vi "Channel List to Pins.vi"(0 "Channel List":string) -> (4 "Sites and Pins":string[](array[string]), 6 "Pins":tag[](array[tag]), 8 "Sites":i32[](array[numeric]))   [LabVIEW 2019]
uses:
  <vilib>/Utility/error.llb/whitespace.ctl
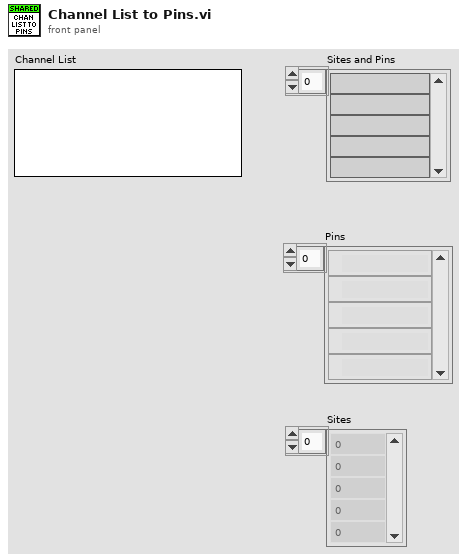
[diagram p1: front panel]
types:
  T1 = typedef "whitespace.ctl" = u16
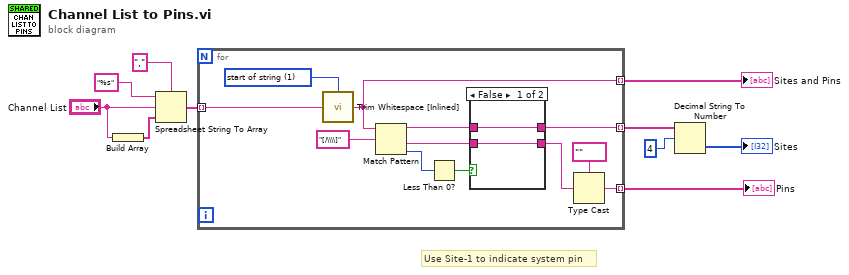
[diagram p0: block diagram]
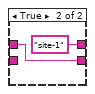
[diagram p2: hidden frame]
diagram:
  # "Use Site-1 to indicate system pin"
  n1 = Build Array("Channel List") -> (w7:string[])
  n2 = Spreadsheet String To Array(delimiter (Tab)=",", format string="%s", spreadsheet string="Channel List", array type (2D Dbl)=w7) -> (array=w6:string[])
  n3 = for {
    tunnel: w6 -> [w22] mode=indexing
    tunnel: [w14] -> w5 mode=indexing
    tunnel: [w19] -> w4 mode=indexing
    tunnel: [w11] -> w1 mode=indexing
    w21 = T1 1 items=["both", "start of string", "end of string"] ("location (both)")
    n4 = call "Trim Whitespace [Inlined].vi"("string"=w22, "location (both)"=w21) -> ("trimmed string"=w19:string)
    n5 = Match Pattern(string=w19, regular expression="[/\\\\]" ("search string/char (-)")) -> (before substring=w15:string, after substring=w16:string, offset past match=w18:i32)  [unwired: 1 in, 1 out]
    n6 = Less Than 0?(x=w18) -> (x < 0?=w17:bool)
    n7 = case shown="False" w17 {
      tunnel: w16 -> [w23 _]
      tunnel: w15 -> [w24 w26]
      tunnel: [w24 "site-1" ("trimmed string")] -> w14
      tunnel: [w23 w26] -> w13
      frame False {
      }
      frame True {
      }
    }
    n8 = Type Cast(type=tag "" ("Pins"), x=w13) -> (*(type *) &x=w11:tag)
  }
  "Pins" <- w1
  "Sites and Pins" <- w4
  n9 = Decimal String To Number(string=w5, offset=4) -> (number=→"Sites":i32[])  [unwired: 1 in, 1 out]
